vi "readFromXML.vi"(8 "error in (no error)":errorcluster, 10 "XML in":string, 11 "RotatorOffsetCommands in":refnum<class "RotatorOffsetCommands.lvclass">) -> (0 "error out":errorcluster, 3 "RotatorOffsetCommands out":refnum<class "RotatorOffsetCommands.lvclass">)   [LabVIEW 2022 SP3, in "TCSDataDefinitions.lvlib" / "TCSCommand.lvlib" / "OffsetCommands.lvlib" / "RotatorOffsetCommands.lvclass"]
uses:
  RotatorOffsetCommands.lvclass
  OffsetCommands/OffsetCommands.lvclass
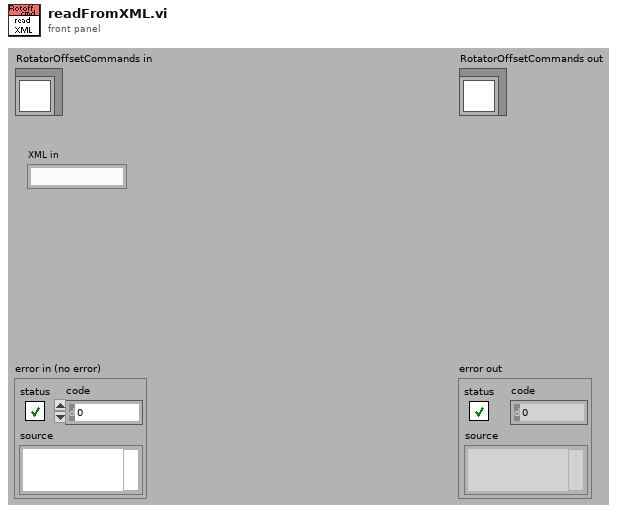
[diagram p1: front panel]
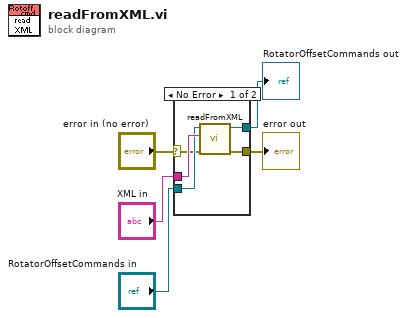
[diagram p0: block diagram]
diagram:
  n1 = case shown="No Error" "error in (no error)" {
    selector: "error in (no error)" -> [w6 w12]
    tunnel: [w10 w12] -> w5
    tunnel: [w9 w11] -> w4
    tunnel: "XML in" -> [w8 _]
    tunnel: "RotatorOffsetCommands in" -> [w7 w11]
    frame No Error {
      n2 = call-parent "readFromXML.vi"("error in (no error)"=w6, "XML in"=w8, "OffsetCommands in"=w7) -> ("error out"=w10:errorcluster, "OffsetCommands out"=w9:refnum<class "RotatorOffsetCommands.lvclass">)  [unwired: 7 out]
    }
    frame Error {
    }
  }
  "error out" <- w5
  "RotatorOffsetCommands out" <- w4
